vi "Cal_Res Table.vi"(2 "Error In":errorcluster, 3 "Action":T1, 4 "Parameters In":T2={"Calibrations"={"Q1 +ve"=[[0.0, 0.0], [59.06, 8007.972231628852], [175.13, 24051.118700948115], [609.3, 84085.25564675158], [616.46, 85075.93195639057], [906.67, 125230.14589777726], [1254.9, 173425.601618889], [1487.09, 205562.74183429], [1500.0, 207349.59949474406]], "Q2 +ve"=[[0.0, 0.0], [59.06, 8023.934304097528], [175.13, 24094.827090057508], [609.3, 84237.75059685535], [616.46, 85258.85953842459], [906.67, 125438.18017005036], [1254.9, 173704.72880677812], [1487.0, 205896.72157687077], [1500.0, 207852.79226600614]], "Q1 -ve"=[[0.0, 0.0], [45.0, 6058.0], [514.1, 70943.72007379876], [585.4, 80765.52138069598], [933.6, 128993.0], [1223.8, 169105.4900068918], [1456.0, 201276.0], [1500.0, 207372.04840524014]], "Q2 -ve"=[[0.0, 0.0], [45.0, 6064.168025288581], [514.1, 71104.0], [585.4, 80965.0], [933.6, 129151.03618609994], [1223.8, 169370.96671193905], [1456.0, 201691.0], [1500.0, 207815.38184614418]]}, "Resolution Q1"={"High +ve"=[[0.0, 33265.24137931035], [59.06, 33900.54299922501], [175.13, 34950.975], [609.3, 38001.81208053691], [616.46, 38045.06040268456], [906.67, 39798.0067114094], [1254.9, 41899.39655117602], [1487.09, 43401.38461538462], [1500.0, 43600.0]], "Med +ve"=[[0.0, 33265.24137931035], [59.06, 33900.54299922501], [175.13, 34950.975], [609.3, 38001.81208053691], [616.46, 38045.06040268456], [906.67, 39798.0067114094], [1254.9, 41899.39655117602], [1487.09, 43401.38461538462], [1500.0, 43600.0]], "Low +ve"=[[0.0, 33265.24137931035], [59.06, 33900.54299922501], [175.13, 34950.975], [609.3, 38001.81208053691], [616.46, 38045.06040268456], [906.67, 39798.0067114094], [1254.9, 41899.39655117602], [1487.09, 43401.38461538462], [1500.0, 43600.0]], "High -ve"=[[0.0, 33265.24137931035], [45.0, 33749.379310344826], [514.1, 37400.0], [585.4, 37795.114503816796], [933.6, 39960.51724137931], [1223.8, 41711.724137931036], [1456.0, 43201.15291898124], [1500.0, 43600.0]], "Med -ve"=[[0.0, 33265.24137931035], [45.0, 33749.379310344826], [514.1, 37400.0], [585.4, 37795.114503816796], [933.6, 39960.51724137931], [1223.8, 41711.724137931036], [1456.0, 43201.15291898124], [1500.0, 43600.0]], "Low -ve"=[[0.0, 33265.24137931035], [45.0, 33749.379310344826], [514.1, 37400.0], [585.4, 37795.114503816796], [933.6, 39960.51724137931], [1223.8, 41711.724137931036], [1456.0, 43201.15291898124], [1500.0, 43600.0]]}, "Resolution Q2"={"High +ve"=[[0.0, 32600.0], [59.06, 33100.0], [175.13, 34050.0], [609.3, 36901.76174496644], [616.46, 36943.80872483221], [906.67, 38648.06208053691], [1254.9, 40749.39656707161], [1487.0, 42150.0], [1500.0, 42300.0]], "Med +ve"=[[0.0, 32600.0], [59.06, 33100.0], [175.13, 34050.0], [609.3, 36901.76174496644], [616.46, 36943.80872483221], [906.67, 38648.06208053691], [1254.9, 40749.39656707161], [1487.0, 42150.0], [1500.0, 42300.0]], "Low +ve"=[[0.0, 32500.0], [45.0, 33050.0], [514.1, 36000.77464788732], [585.4, 36552.29226361032], [933.6, 38547.70773638968], [1223.8, 40148.896492931395], [1456.0, 41430.06819957849], [1500.0, 41672.83975467096]], "High -ve"=[[0.0, 32500.0], [45.0, 33050.0], [514.1, 36000.77464788732], [585.4, 36552.29226361032], [933.6, 38547.70773638968], [1223.8, 40148.896492931395], [1456.0, 41430.06819957849], [1500.0, 41672.83975467096]], "Med -ve"=[[0.0, 32500.0], [45.0, 33050.0], [514.1, 36000.77464788732], [585.4, 36552.29226361032], [933.6, 38547.70773638968], [1223.8, 40148.896492931395], [1456.0, 41430.06819957849], [1500.0, 41672.83975467096]], "Low -ve"=[[0.0, 32500.0], [45.0, 33050.0], [514.1, 36000.77464788732], [585.4, 36552.29226361032], [933.6, 38547.70773638968], [1223.8, 40148.896492931395], [1456.0, 41430.06819957849], [1500.0, 41672.83975467096]]}} {"Resolution Q2"."Low -ve" format="%.2f"; "Resolution Q2"."Med -ve" format="%.2f"; "Resolution Q2"."High -ve" format="%.2f"; "Resolution Q2"."Low +ve" format="%.2f"; "Resolution Q2"."Med +ve" format="%.2f"; "Resolution Q2"."High +ve" format="%.2f"; "Resolution Q1"."Low -ve" format="%.2f"; "Resolution Q1"."Med -ve" format="%.2f"; "Resolution Q1"."High -ve" format="%.2f"; "Resolution Q1"."Low +ve" format="%.2f"; "Resolution Q1"."Med +ve" format="%.2f"; "Resolution Q1"."High +ve" format="%.2f"; "Calibrations"."Q2 -ve" format="%.2f"; "Calibrations"."Q1 -ve" format="%.2f"; "Calibrations"."Q2 +ve" format="%.2f"; "Calibrations"."Q1 +ve" format="%.2f"}) -> (0 "Error Out":errorcluster, 1 "Parameters Out":T2={"Calibrations"={"Q1 +ve"=[[0.0, 0.0], [59.06, 8007.972231628852], [175.13, 24051.118700948115], [609.3, 84085.25564675158], [616.46, 85075.93195639057], [906.67, 125230.14589777726], [1254.9, 173425.601618889], [1487.09, 205562.74183429], [1500.0, 207349.59949474406]], "Q2 +ve"=[[0.0, 0.0], [59.06, 8023.934304097528], [175.13, 24094.827090057508], [609.3, 84237.75059685535], [616.46, 85258.85953842459], [906.67, 125438.18017005036], [1254.9, 173704.72880677812], [1487.0, 205896.72157687077], [1500.0, 207852.79226600614]], "Q1 -ve"=[[0.0, 0.0], [45.0, 6058.0], [514.1, 70943.72007379876], [585.4, 80765.52138069598], [933.6, 128993.0], [1223.8, 169105.4900068918], [1456.0, 201276.0], [1500.0, 207372.04840524014]], "Q2 -ve"=[[0.0, 0.0], [45.0, 6064.168025288581], [514.1, 71104.0], [585.4, 80965.0], [933.6, 129151.03618609994], [1223.8, 169370.96671193905], [1456.0, 201691.0], [1500.0, 207815.38184614418]]}, "Resolution Q1"={"High +ve"=[[0.0, 33265.24137931035], [59.06, 33900.54299922501], [175.13, 34950.975], [609.3, 38001.81208053691], [616.46, 38045.06040268456], [906.67, 39798.0067114094], [1254.9, 41899.39655117602], [1487.09, 43401.38461538462], [1500.0, 43600.0]], "Med +ve"=[[0.0, 33265.24137931035], [59.06, 33900.54299922501], [175.13, 34950.975], [609.3, 38001.81208053691], [616.46, 38045.06040268456], [906.67, 39798.0067114094], [1254.9, 41899.39655117602], [1487.09, 43401.38461538462], [1500.0, 43600.0]], "Low +ve"=[[0.0, 33265.24137931035], [59.06, 33900.54299922501], [175.13, 34950.975], [609.3, 38001.81208053691], [616.46, 38045.06040268456], [906.67, 39798.0067114094], [1254.9, 41899.39655117602], [1487.09, 43401.38461538462], [1500.0, 43600.0]], "High -ve"=[[0.0, 33265.24137931035], [45.0, 33749.379310344826], [514.1, 37400.0], [585.4, 37795.114503816796], [933.6, 39960.51724137931], [1223.8, 41711.724137931036], [1456.0, 43201.15291898124], [1500.0, 43600.0]], "Med -ve"=[[0.0, 33265.24137931035], [45.0, 33749.379310344826], [514.1, 37400.0], [585.4, 37795.114503816796], [933.6, 39960.51724137931], [1223.8, 41711.724137931036], [1456.0, 43201.15291898124], [1500.0, 43600.0]], "Low -ve"=[[0.0, 33265.24137931035], [45.0, 33749.379310344826], [514.1, 37400.0], [585.4, 37795.114503816796], [933.6, 39960.51724137931], [1223.8, 41711.724137931036], [1456.0, 43201.15291898124], [1500.0, 43600.0]]}, "Resolution Q2"={"High +ve"=[[0.0, 32600.0], [59.06, 33100.0], [175.13, 34050.0], [609.3, 36901.76174496644], [616.46, 36943.80872483221], [906.67, 38648.06208053691], [1254.9, 40749.39656707161], [1487.0, 42150.0], [1500.0, 42300.0]], "Med +ve"=[[0.0, 32600.0], [59.06, 33100.0], [175.13, 34050.0], [609.3, 36901.76174496644], [616.46, 36943.80872483221], [906.67, 38648.06208053691], [1254.9, 40749.39656707161], [1487.0, 42150.0], [1500.0, 42300.0]], "Low +ve"=[[0.0, 32500.0], [45.0, 33050.0], [514.1, 36000.77464788732], [585.4, 36552.29226361032], [933.6, 38547.70773638968], [1223.8, 40148.896492931395], [1456.0, 41430.06819957849], [1500.0, 41672.83975467096]], "High -ve"=[[0.0, 32500.0], [45.0, 33050.0], [514.1, 36000.77464788732], [585.4, 36552.29226361032], [933.6, 38547.70773638968], [1223.8, 40148.896492931395], [1456.0, 41430.06819957849], [1500.0, 41672.83975467096]], "Med -ve"=[[0.0, 32500.0], [45.0, 33050.0], [514.1, 36000.77464788732], [585.4, 36552.29226361032], [933.6, 38547.70773638968], [1223.8, 40148.896492931395], [1456.0, 41430.06819957849], [1500.0, 41672.83975467096]], "Low -ve"=[[0.0, 32500.0], [45.0, 33050.0], [514.1, 36000.77464788732], [585.4, 36552.29226361032], [933.6, 38547.70773638968], [1223.8, 40148.896492931395], [1456.0, 41430.06819957849], [1500.0, 41672.83975467096]]}} {"Resolution Q2"."Low -ve" format="%.2f"; "Resolution Q2"."Med -ve" format="%.2f"; "Resolution Q2"."High -ve" format="%.2f"; "Resolution Q2"."Low +ve" format="%.2f"; "Resolution Q2"."Med +ve" format="%.2f"; "Resolution Q2"."High +ve" format="%.2f"; "Resolution Q1"."Low -ve" format="%.2f"; "Resolution Q1"."Med -ve" format="%.2f"; "Resolution Q1"."High -ve" format="%.2f"; "Resolution Q1"."Low +ve" format="%.2f"; "Resolution Q1"."Med +ve" format="%.2f"; "Resolution Q1"."High +ve" format="%.2f"; "Calibrations"."Q2 -ve" format="%.2f"; "Calibrations"."Q1 -ve" format="%.2f"; "Calibrations"."Q2 +ve" format="%.2f"; "Calibrations"."Q1 +ve" format="%.2f"})   [LabVIEW 2018]
uses:
  Type Defs/CAL_RES.ctl
  Type Defs/Global Action.ctl
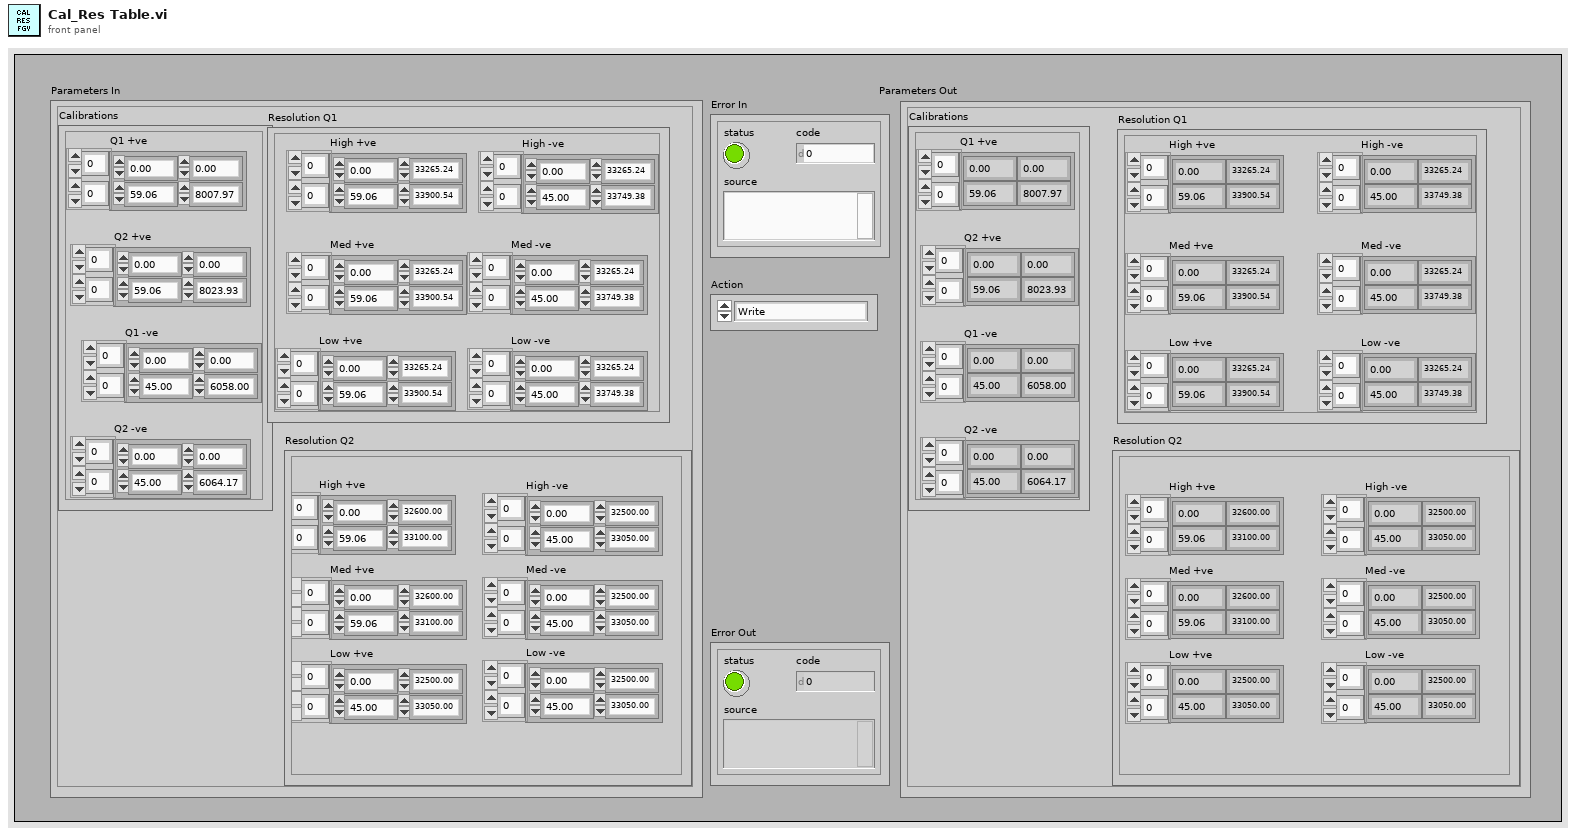
[diagram p1: front panel]
types:
  T1 = typedef "Global Action.ctl" = enum16{"Write", "Read"}
  T2 = typedef "CAL_RES.ctl" = cluster{"Calibrations":cluster{"Q1 +ve":dbl[][], "Q2 +ve":dbl[][], "Q1 -ve":dbl[][], "Q2 -ve":dbl[][]}, "Resolution Q1":cluster{"High +ve":dbl[][], "Med +ve":dbl[][], "Low +ve":dbl[][], "High -ve":dbl[][], "Med -ve":dbl[][], "Low -ve":dbl[][]}, "Resolution Q2":cluster{"High +ve":dbl[][], "Med +ve":dbl[][], "Low +ve":dbl[][], "High -ve":dbl[][], "Med -ve":dbl[][], "Low -ve":dbl[][]}}
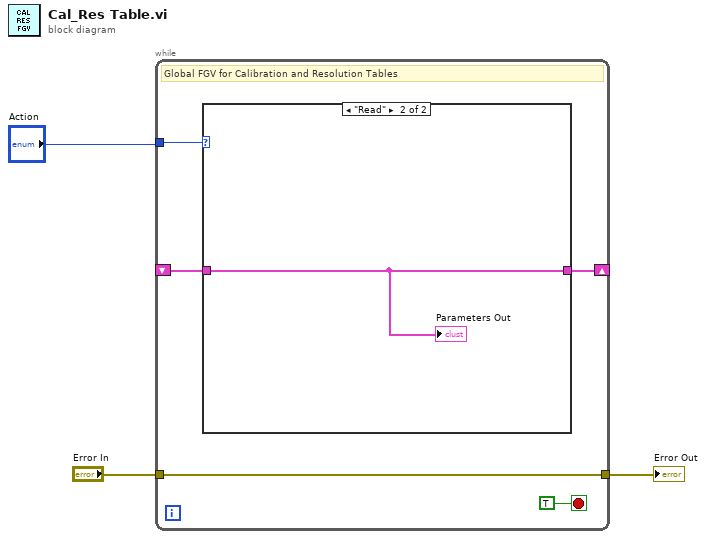
[diagram p0: block diagram]
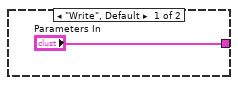
[diagram p2: hidden frame]
diagram:
  n1 = while {
    tunnel: "Action" -> [w7]
    tunnel: "Error In" -> [w6]
    tunnel: [w6] -> w1
    shift-right: [w5] -> _
    shift-left: _ -> [w4]
    stop <- TRUE stop-if-true
    # "Global FGV for Calibration and Resolution Tables"
    n2 = case shown="\"Read\"" w7 {
      tunnel: ["Parameters In" w10] -> w5
      tunnel: w4 -> [_ w10]
      frame "Write", Default {
      }
      frame "Read" {
        "Parameters Out" <- w10
      }
    }
  }
  "Error Out" <- w1
